vi "operation.vi"(1 "Input 2":dbl, 2 "Operator":string(combo), 3 "Input 1":dbl) -> (0 "Numeric":dbl)   [LabVIEW 2011]
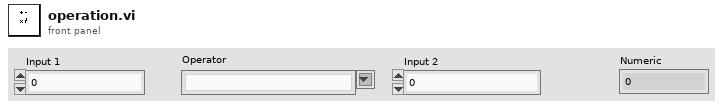
[diagram p1: front panel]
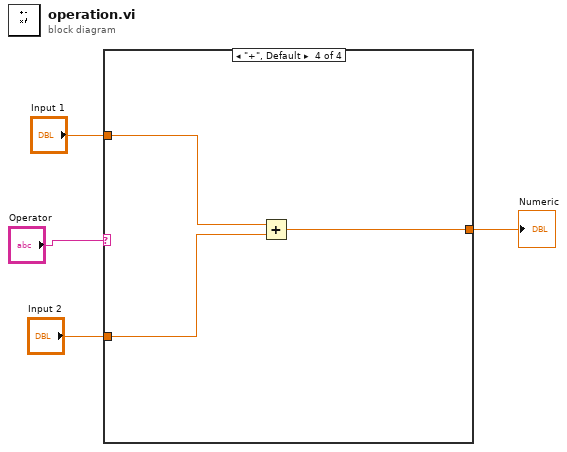
[diagram p0: block diagram]
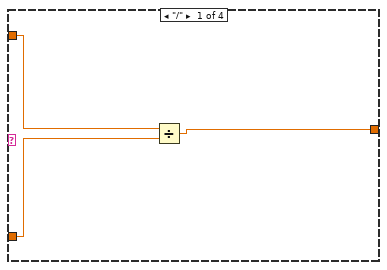
[diagram p2: hidden frame]
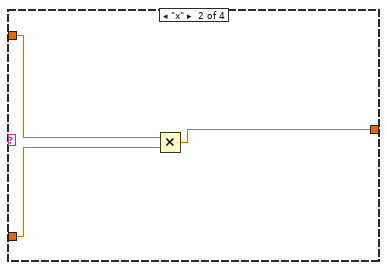
[diagram p3: hidden frame]
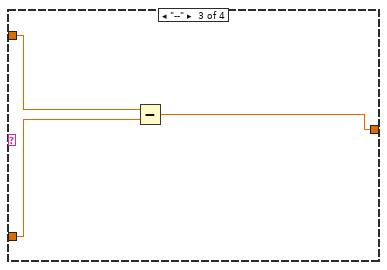
[diagram p4: hidden frame]
diagram:
  n1 = case shown="\"+\", Default" "Operator" {
    tunnel: "Input 1" -> [w7 w10 w13 w16]
    tunnel: "Input 2" -> [w6 w9 w12 w15]
    tunnel: [w5 w8 w11 w14] -> w1
    frame "/" {
      n2 = Divide(x=w7, y=w6) -> (x/y=w5:dbl)
    }
    frame "x" {
      n3 = Multiply(x=w10, y=w9) -> (x*y=w8:dbl)
    }
    frame "--" {
      n4 = Subtract(x=w13, y=w12) -> (x-y=w11:dbl)
    }
    frame "+", Default {
      n5 = Add(x=w16, y=w15) -> (x+y=w14:dbl)
    }
  }
  "Numeric" <- w1
